vi "DHE_Lib_integrate.vi"(7 "msecs":u32, 11 "error in (no error)":errorcluster) -> (8 "return value":i32, 10 "dark time":i32, 15 "error out":errorcluster)   [LabVIEW 2016]
doc: "This VI opens (Flag=1) or closes (Flag=0) the instrument shutter."
uses:
  c/lib/libgendhe.so
panel:
  in  "dark":i32
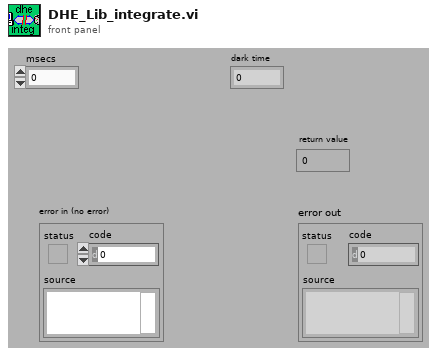
[diagram p1: front panel]
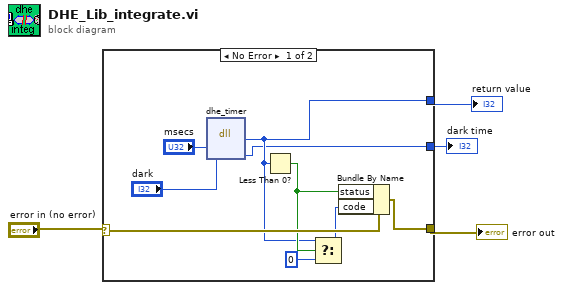
[diagram p0: block diagram]
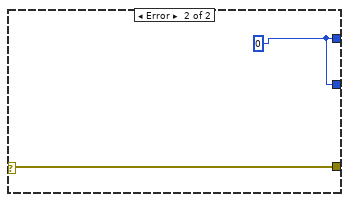
[diagram p2: hidden frame]
diagram:
  n1 = case shown="No Error" "error in (no error)" {
    selector: "error in (no error)" -> [w12 w15]
    tunnel: [w11 w15] -> w4
    tunnel: [w9 w14] -> w2
    tunnel: [w5 w14] -> w1
    frame No Error {
      n2 = dll-call lib="home/sispi/panview/PAN/Modules/DHE/private/c/lib/libgendhe.so" fn="dhe_timer"("msecs"="msecs", "darktime"="dark") -> ("return type"=w9:i32, "darktime"=w5:i32)  [unwired: 4 in, 2 out]
      n3 = Less Than 0?(x=w9) -> (x < 0?=w10:bool)
      n4 = Select(t=w9, s=w10, f=0) -> (s? t:f=w8:i32)
      n5 = Bundle By Name(cluster=w12, "status"=w10, "code"=w8) -> (w11:errorcluster)
    }
    frame Error {
      w14 = 0
    }
  }
  "error out" <- w4
  "return value" <- w2
  "dark time" <- w1
